vi "FTW-Actor-Core-SpawnPrelude.vi"(5 "Actor Instance Configuration":string="{\n  \"Identity\": \"ActorName\",\n  \"InboxAddress\": \"tcp://127.0.0.1:*\",\n  \"SupervisorAddress\": \"\",\n  \"DebugEnableInboxLogging\": false,\n  \"DebugEnableJobLogging\": false,\n  \"DebugShowPanel\": false\n}", 11 "error in":errorcluster) -> (4 "Spawn Options":T1={"HandshakeTimeout"=2000, "Handshaker"=refnum, "ShowPanelSpecified"=TRUE, "ShowPanelValue"=TRUE} {"HandshakeTimeout" format="%d msec"}, 6 "Actor Instance Configuration out":string, 15 "error out":errorcluster)   [LabVIEW 2015]
uses:
  FTW-Actor-Core-SpawnOptions.ctl
  core/type/FTW-Type-JSON.ctl
  json/FTW-JSON-Type.ctl
  json/core/FTW-JSON-Core-Type.ctl
  lib/FTW-KernelFilepath.vi
  json/core/FTW-JSON-Core-LibraryReturnValue.vi
  error/FTW-ERR-ThrowInvalidReferenceError.vi
  json/core/FTW-JSON-Core-ElementType.vi
  codegen/xnode/FTW-JSON-Fetch.xnode
panel:
  # "Inputs"
  # "Outputs"
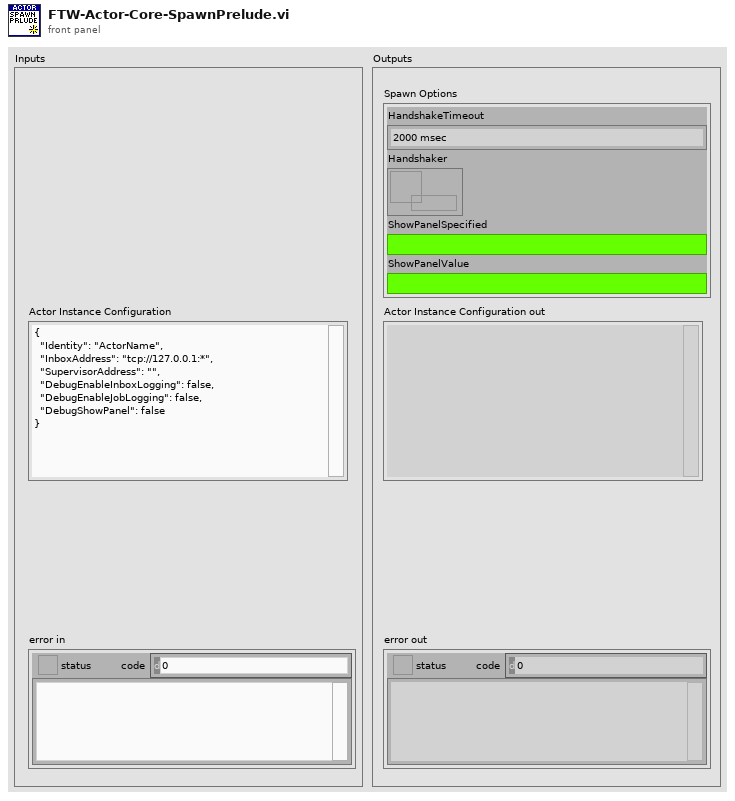
[diagram p1: front panel]
types:
  T1 = typedef "FTW-Actor-Core-SpawnOptions.ctl" = cluster{"HandshakeTimeout":i32, "Handshaker":refnum<queue>, "ShowPanelSpecified":bool, "ShowPanelValue":bool}
  T2 = typedef "FTW-JSON-Type.ctl" = enum8{"Not Found", "Object", "Array", "String", "Number", "Boolean", "null"}
  T3 = typedef "FTW-Type-JSON.ctl" = refnum<data-value>
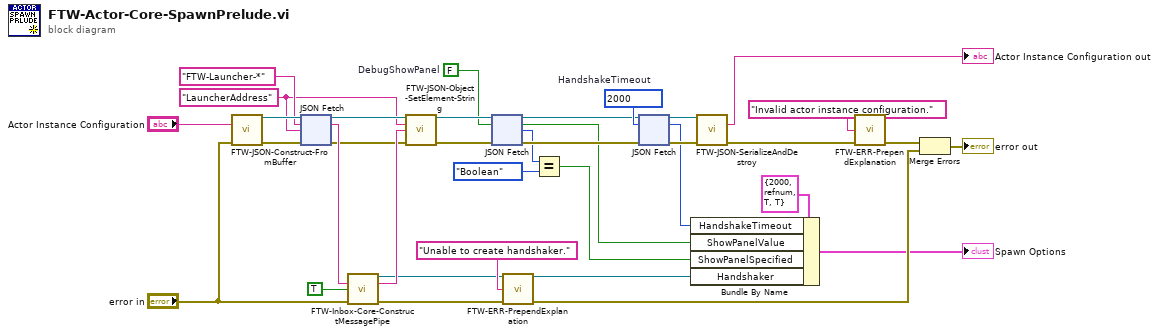
[diagram p0: block diagram]
diagram:
  w19 = FALSE  # DebugShowPanel
  w17 = 2000  # HandshakeTimeout
  w21 = "LauncherAddress" ("Key")
  n1 = call "FTW-JSON-Construct-FromBuffer.vi"("JSON String (UTF-8)"="Actor Instance Configuration", "error in"="error in") -> ("JSON"=w27:T3, "error out"=w23:errorcluster)  [unwired: 12 in]
  n2 = xnode "JSON Fetch"("JSON"=w27, "Element Type and Default Value"="FTW-Launcher-*" ("Actor Identity (empty to create unnamed actor)"), "Element Path"=w21, "error in"=w23) -> ("JSON out"=w26:T3, "Value"=w24:string, "error out"=w22:errorcluster)  [unwired: 1 in, 1 out]
  n3 = call "FTW-Inbox-Core-ConstructMessagePipe.vi"("Actor Identity (empty to create unnamed actor)"=w24, "Is Primary?"=TRUE, "error in"="error in") -> ("Message Pipe"=w8:refnum<queue>, "Resolved Actor Identity"=w29:string, "error out"=w30:errorcluster)  [unwired: 10 in]
  n4 = call "FTW-JSON-Object-SetElement-String.vi"("JSON"=w26, "Key"=w21, "Value"=w29, "error in"=w22) -> ("JSON out"=w20:T3, "error out"=w18:errorcluster)  [unwired: 10 in]
  n5 = xnode "JSON Fetch"("JSON"=w20, "Element Type and Default Value"=w19, "error in"=w18) -> ("JSON out"=w16:T3, "Value"=w4:bool, "JSON Element Type"=w6:T2, "error out"=w14:errorcluster)  [unwired: 2 in]
  n6 = call "FTW-ERR-PrependExplanation.vi"("Exception Information"="Unable to create handshaker.", "error in"=w30) -> ("error out"=w35:errorcluster)  [unwired: 13 in]
  n7 = Equal?(x=w6, y=FTW-JSON-Type."Boolean" ("JSON Element Type")) -> (x = y?=w3:bool)
  n8 = xnode "JSON Fetch"("JSON"=w16, "Element Type and Default Value"=w17, "error in"=w14) -> ("JSON out"=w15:T3, "Value"=w9:i32, "error out"=w13:errorcluster)  [unwired: 2 in, 1 out]
  n9 = Bundle By Name(cluster=T1 {"HandshakeTimeout"=2000, "Handshaker"=refnum, "ShowPanelSpecified"=TRUE, "ShowPanelValue"=TRUE} ("Spawn Options"), "HandshakeTimeout"=w9, "ShowPanelValue"=w4, "ShowPanelSpecified"=w3, "Handshaker"=w8) -> (→"Spawn Options":T1)
  n10 = call "FTW-JSON-SerializeAndDestroy.vi"("JSON"=w15, "error in"=w13) -> ("JSON String (UTF-8)"=→"Actor Instance Configuration out":string, "error out"=w33:errorcluster)  [unwired: 12 in]
  n11 = call "FTW-ERR-PrependExplanation.vi"("Exception Information"="Invalid actor instance configuration.", "error in"=w33) -> ("error out"=w32:errorcluster)  [unwired: 13 in]
  n12 = Merge Errors(w32, w35) -> (→"error out":errorcluster)
